vi "Receive UDP.vi"(6 "Operation":enum16{"Init", "Receive", "Close"}(ring)=enum."Receive", 8 "error in":errorcluster, 11 "receiver port":u16=61557) -> (0 "error out":errorcluster, 1 "O Data":dbl[](array[numeric]), 2 "Data":i32)   [LabVIEW 2021]
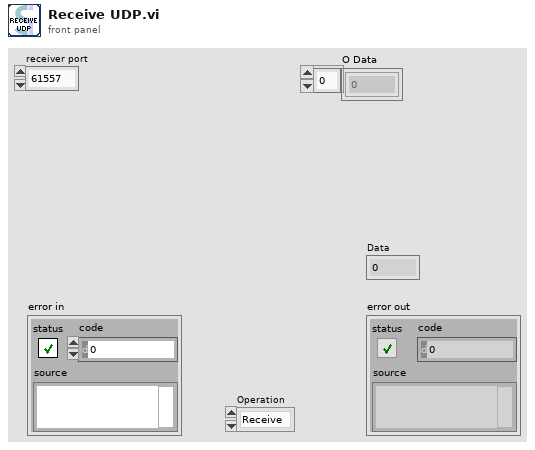
[diagram p1: front panel]
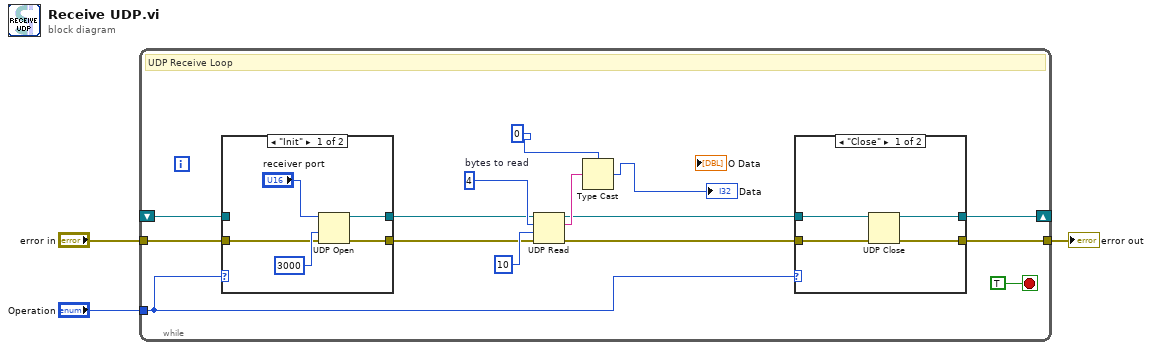
[diagram p0: block diagram]
diagram:
  n1 = while {
    tunnel: "error in" -> [w17]
    shift-right: [w14] -> _
    shift-left: _ -> [w16]
    tunnel: "Operation" -> [w6]
    tunnel: [w15] -> w1
    stop <- TRUE stop-if-true
    w12 = 4  # bytes to read
    # "UDP Receive Loop"
    n2 = case shown="\"Init\"" w6 {
      tunnel: w17 -> [w25 w30]
      tunnel: [w28 w30] -> w7
      tunnel: [w27 w31] -> w8
      tunnel: w16 -> [_ w31]
      frame "Init" {
        n3 = UDP Open(8:w25, 9:3000 ("timeout ms (25000)"), 11:"receiver port") -> (port=w27:refnum<k16>, 0:w28:errorcluster)  [unwired: 2 in, 1 out]
      }
      frame "Receive", Default {
      }
    }
    n4 = UDP Read(connection ID=w8, max size (548)=w12, timeout ms (25000)=10, 8:w7) -> (data out=w13:string, error out=w11:errorcluster, 3:w9:refnum<k16>)  [unwired: 2 out]
    n5 = Type Cast(type=0 ("Data"), x=w13) -> (*(type *) &x=→"Data":i32)
    n6 = case shown="\"Close\"" w6 {
      tunnel: w11 -> [w22 w24]
      tunnel: [w21 w24] -> w15
      tunnel: w9 -> [w20 w23]
      tunnel: [w19 w23] -> w14
      frame "Close" {
        n7 = UDP Close(connection ID=w20, 8:w22) -> (connection ID out=w19:refnum<k16>, error out=w21:errorcluster)
      }
      frame "Receive", Default {
      }
    }
  }
  "error out" <- w1
